vi "Auto_LL_Shoot.vi"(10 "Boolean":bool) -> ()   [LabVIEW 2019]
uses:
  <vilib>/Rock Robotics/Network Tables/NT Write Number.vi
  <vilib>/Rock Robotics/Network Tables/NT Read Number.vi
  <vilib>/Rock Robotics/WPI/RobotDrive/WPI_RobotDriveMecanumDrive_Cartesian.vi
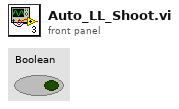
[diagram p1: front panel]
types:
  T1 = typedef "WPI_MotorControlDeviceRef.ctl" = cluster{"DeviceStatus":errorcluster, "Type":T2, "PWM":cluster{"PWM Channel":T3, "DeadBand":T4}, "CAN":cluster{"Device Number":u8, "SetOutput VI Ref":variant, "GetOutput VI Ref":variant, "Enable VI Ref":variant, "Disable VI Ref":variant, "Data":variant}, "Invert":bool, "DIO PWM":cluster{"PWM \"Enable\" Channel":T3, "DIOChannel":T5, "PWM Rate":dbl}}
  T2 = typedef "WPI_MotorControlType.ctl" = enum16{"PWM", "CAN", "DIO PWM"}
  T3 = typedef "FPGA_DIOPWMChannel.ctl" = enum8{"PWM 0", "PWM 1", "PWM 2", "PWM 3", "PWM 4", "PWM 5", "PWM 6", "PWM 7", "PWM 8", "PWM 9", "PWM MXP 0", "PWM MXP 1", "PWM MXP 2", "PWM MXP 3", "PWM MXP 4", "PWM MXP 5", "PWM MXP 6", "PWM MXP 7", "PWM MXP 8", "PWM MXP 9", "Invalid"}
  T4 = typedef "WPI_PWMDeadband.ctl" = cluster{"Name":string, "maxPositivePwm":i32, "minPositivePwm":i32, "centerPwm":i32, "maxNegativePwm":i32, "minNegativePwm":i32, "angularRange":u16}
  T5 = typedef "FPGA_DIOChannel.ctl" = enum8{"DIO 0", "DIO 1", "DIO 2", "DIO 3", "DIO 4", "DIO 5", "DIO 6", "DIO 7", "DIO 8", "DIO 9", "DIO MXP 0", "DIO MXP 1", "DIO MXP 2", "DIO MXP 3", "DIO MXP 4", "DIO MXP 5", "DIO MXP 6", "DIO MXP 7", "DIO MXP 8", "DIO MXP 9", "DIO MXP 10", "DIO MXP 11", "DIO MXP 12", "DIO MXP 13", "DIO MXP 14", "DIO MXP 15", "SPI Port CS1", "SPI Port CS2", "SPI Port CS3", "SPI Port MISO", "SPI Port MOSI", "Invalid"}
  T6 = typedef "WPI_RobotDriveDevRef.ctl" = cluster{"DevStatus":errorcluster, "Motors[]":T1[], "Square Inputs":bool, "Max Output":dbl}
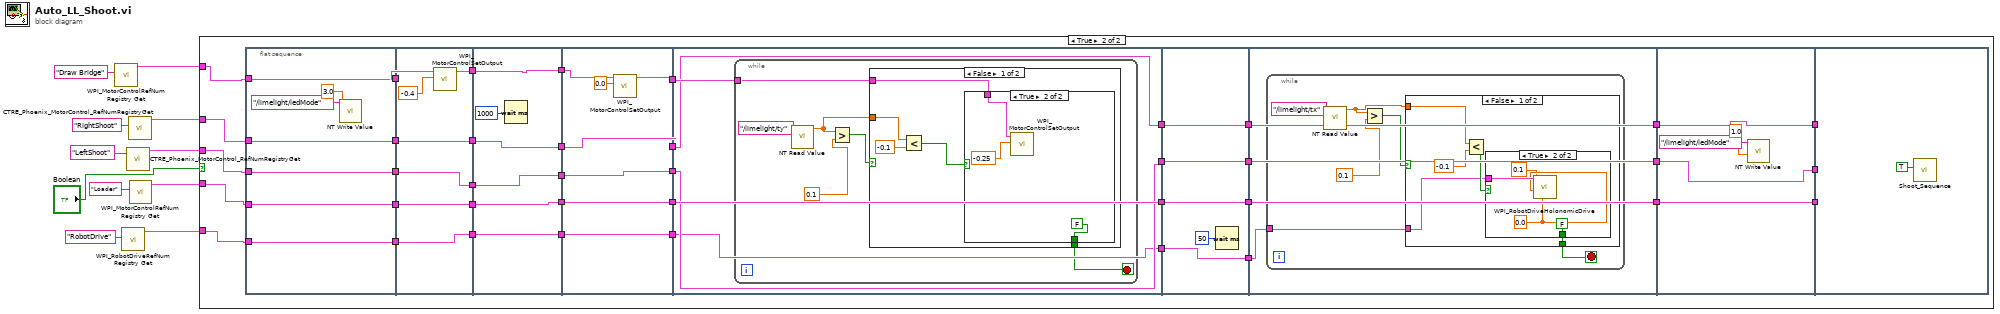
[diagram p0: block diagram]
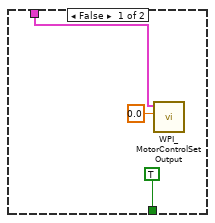
[diagram p3: hidden frame]
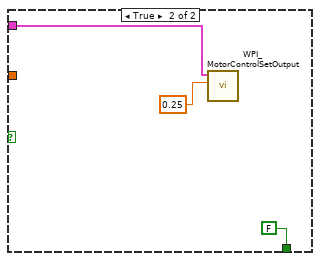
[diagram p4: hidden frame]
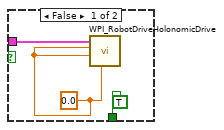
[diagram p5: hidden frame]
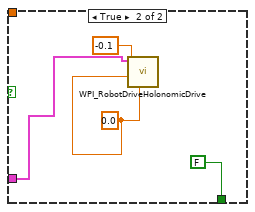
[diagram p6: hidden frame]
diagram:
  n1 = call <vilib>:"WPI_MotorControlRefNum Registry Get.vi"("refnum name"="Draw Bridge") -> ("MotorControlDevRef"=w7:T1)  [unwired: 9 in, 1 out]
  n2 = call <vilib>:"WPI_RobotDriveRefNum Registry Get.vi"("refnum name"="RobotDrive") -> ("RobotDriveDevRef"=w2:T6)  [unwired: 9 in, 1 out]
  n3 = call <vilib>:"CTRE_Phoenix_MotorControl_RefNumRegistryGet.vi"("refnum name"="LeftShoot") -> ("PhoenixMotorControlDevRef"=w4:T1)  [unwired: 9 in, 1 out]
  n4 = call <vilib>:"CTRE_Phoenix_MotorControl_RefNumRegistryGet.vi"("refnum name"="RightShoot") -> ("PhoenixMotorControlDevRef"=w5:T1)  [unwired: 9 in, 1 out]
  n5 = call <vilib>:"WPI_MotorControlRefNum Registry Get.vi"("refnum name"="Loader") -> ("MotorControlDevRef"=w3:T1)  [unwired: 9 in, 1 out]
  n6 = case shown="True" "Boolean" {
    tunnel: w7 -> [_ w16]
    tunnel: w5 -> [_ w15]
    tunnel: w4 -> [_ w14]
    tunnel: w3 -> [_ w13]
    tunnel: w2 -> [_ w12]
    frame False {
    }
    frame True {
      n7 = flat-sequence {
        tunnel: w15 -> [w54]
        tunnel: w14 -> [w55]
        tunnel: w16 -> [w56]
        tunnel: w13 -> [w57]
        tunnel: [w57] -> w50
        tunnel: [w56] -> w49
        tunnel: [w55] -> w48
        tunnel: [w54] -> w47
        tunnel: [w51] -> w46
        tunnel: w12 -> [w51]
        tunnel: [w64] -> w45
        tunnel: [w61] -> w44
        tunnel: [w60] -> w43
        tunnel: [w59] -> w42
        tunnel: w50 -> [w64]
        tunnel: w49 -> [w63]
        tunnel: w48 -> [w60]
        tunnel: w47 -> [w59]
        tunnel: [w58] -> w41
        tunnel: w46 -> [w58]
        tunnel: [w70] -> w37
        tunnel: w45 -> [w70]
        tunnel: w44 -> [w69]
        tunnel: [w69] -> w38
        tunnel: [w67] -> w39
        tunnel: w43 -> [w67]
        tunnel: [w66] -> w40
        tunnel: w42 -> [w66]
        tunnel: [w65] -> w36
        tunnel: w41 -> [w65]
        tunnel: [w77] -> w34
        tunnel: [w76] -> w35
        tunnel: [w75] -> w33
        tunnel: [w74] -> w32
        tunnel: w40 -> [w74]
        tunnel: w39 -> [w75]
        tunnel: w38 -> [w73]
        tunnel: w37 -> [w77]
        tunnel: [w71] -> w31
        tunnel: w36 -> [w71]
        tunnel: [w81] -> w30
        tunnel: w35 -> [w82]
        tunnel: w34 -> [w81]
        tunnel: w33 -> [w79]
        tunnel: w32 -> [w80]
        tunnel: [w80] -> w29
        tunnel: [w79] -> w28
        tunnel: [w78] -> w27
        tunnel: w31 -> [w78]
        tunnel: w30 -> [w107]
        tunnel: [w107] -> w26
        tunnel: w29 -> [w106]
        tunnel: [w106] -> w25
        tunnel: w28 -> [w105]
        tunnel: [w105] -> w24
        tunnel: [w103] -> w23
        tunnel: w27 -> [w103]
        tunnel: w26 -> [w111]
        tunnel: [w111] -> w22
        tunnel: w25 -> [w110]
        tunnel: [w110] -> w21
        tunnel: w24 -> [w109]
        tunnel: [w109] -> w20
        tunnel: w23 -> [w108]
        tunnel: w22 -> [w136]
        tunnel: w21 -> [w134]
        tunnel: w20 -> [w135]
        tunnel: [w136] -> w19
        tunnel: [w135] -> w18
        tunnel: [w134] -> w17
        tunnel: w19 -> [_]
        tunnel: w18 -> [_]
        tunnel: w17 -> [_]
        frame #0 {
          n8 = call-poly <vilib>:"NT Write Value.vi"("Numeric"=3.0, "Name"="/limelight/ledMode") -> ()  [unwired: 9 in, 1 out]
        }
        frame #1 {
          n9 = call <vilib>:"WPI_MotorControlSetOutput.vi"("Output"=-0.4, "MotorControlDevRef"=w63) -> ("MotorControlDevRef"=w61:T1)  [unwired: 7 in, 2 out]
        }
        frame #2 {
          n10 = Wait (ms)(milliseconds to wait=u32 1000) -> ()  [unwired: 1 out]
        }
        frame #3 {
          n11 = call <vilib>:"WPI_MotorControlSetOutput.vi"("Output"=0.0, "MotorControlDevRef"=w73) -> ("MotorControlDevRef"=w76:T1)  [unwired: 7 in, 2 out]
        }
        frame #4 {
          n12 = while {
            tunnel: w82 -> [w85]
            stop <- w83 stop-if-true
            n13 = call-poly <vilib>:"NT Read Value.vi"("Name"="/limelight/ty") -> ("Numeric"=w84:dbl)  [unwired: 9 in, 1 out]
            n14 = Greater?(x=w84, y=0.1) -> (0:w86:bool)
            n15 = case shown="False" w86 {
              tunnel: w84 -> [w92 _]
              tunnel: w85 -> [w90 w101]
              tunnel: [w89 FALSE] -> w83
              frame False {
                n16 = Less?(x=w92, y=-0.1) -> (x < y?=w91:bool)
                n17 = case shown="True" w91 {
                  tunnel: w90 -> [w95 w98]
                  tunnel: [TRUE FALSE] -> w89
                  frame False {
                    n18 = call <vilib>:"WPI_MotorControlSetOutput.vi"("Output"=0.0, "MotorControlDevRef"=w95) -> ()  [unwired: 7 in, 3 out]
                  }
                  frame True {
                    n19 = call <vilib>:"WPI_MotorControlSetOutput.vi"("Output"=-0.25, "MotorControlDevRef"=w98) -> ()  [unwired: 7 in, 3 out]
                  }
                }
              }
              frame True {
                n20 = call <vilib>:"WPI_MotorControlSetOutput.vi"("Output"=0.25, "MotorControlDevRef"=w101) -> ()  [unwired: 7 in, 3 out]
              }
            }
          }
        }
        frame #5 {
          n21 = Wait (ms)(milliseconds to wait=u32 50) -> ()  [unwired: 1 out]
        }
        frame #6 {
          n22 = while {
            tunnel: w108 -> [w113]
            stop <- w112 stop-if-true
            n23 = call-poly <vilib>:"NT Read Value.vi"("Name"="/limelight/tx") -> ("Numeric"=w114:dbl)  [unwired: 9 in, 1 out]
            n24 = Greater?(x=w114, y=0.1) -> (0:w115:bool)
            n25 = case shown="False" w115 {
              tunnel: w114 -> [w120 _]
              tunnel: w113 -> [w119 w133]
              tunnel: [w118 FALSE] -> w112
              frame False {
                n26 = Less?(x=w120, y=-0.1) -> (x < y?=w121:bool)
                n27 = case shown="True" w121 {
                  tunnel: w119 -> [w125 w129]
                  tunnel: [TRUE FALSE] -> w118
                  frame False {
                    w124 = 0.0 ("y")
                    n28 = call-poly <vilib>:"WPI_RobotDriveHolonomicDrive.vi"("Rotation"=w124, "Y"=w124, "X"=w124, "RobotDriveDevRef"=w125) -> ()  [unwired: 5 in, 3 out]
                  }
                  frame True {
                    w128 = 0.0 ("Rotation")
                    n29 = call-poly <vilib>:"WPI_RobotDriveHolonomicDrive.vi"("Rotation"=w128, "Y"=w128, "X"=0.1, "RobotDriveDevRef"=w129) -> ()  [unwired: 5 in, 3 out]
                  }
                }
              }
              frame True {
                w132 = 0.0 ("Rotation")
                n30 = call-poly <vilib>:"WPI_RobotDriveHolonomicDrive.vi"("Rotation"=w132, "Y"=w132, "X"=-0.1, "RobotDriveDevRef"=w133) -> ()  [unwired: 5 in, 3 out]
              }
            }
          }
        }
        frame #7 {
          n31 = call-poly <vilib>:"NT Write Value.vi"("Numeric"=1.0, "Name"="/limelight/ledMode") -> ()  [unwired: 9 in, 1 out]
        }
        frame #8 {
          n32 = call "Shoot_Sequence.vi"("Start?"=TRUE) -> ()  [unwired: 11 in]
        }
      }
    }
  }
